vi "Do.vi"(8 "error in (no error)":errorcluster, 10 "Actor in":refnum<class "Actor.lvclass">, 11 "Items Double Click Msg":refnum<class "Items Double Click Msg.lvclass">) -> (0 "error out":errorcluster, 2 "Actor out":refnum<class "Actor.lvclass">)   [LabVIEW 2016, in "Items Double Click Msg.lvclass"]
doc: "This VI delivers the message to the actor by calling the appropriate method(s) on the actor."
uses:
  Items Double Click Msg.lvclass
  <vilib>/ActorFramework/Actor/Actor.lvclass
  Sequence Element/Sequence Element.lvclass
  D:/Program Files/National Instruments/LabVIEW 2016/vi.lib/ActorFramework/Actor/Actor.lvclass
  Items Double Click Msg.lvclass/Items Double Click Msg.ctl
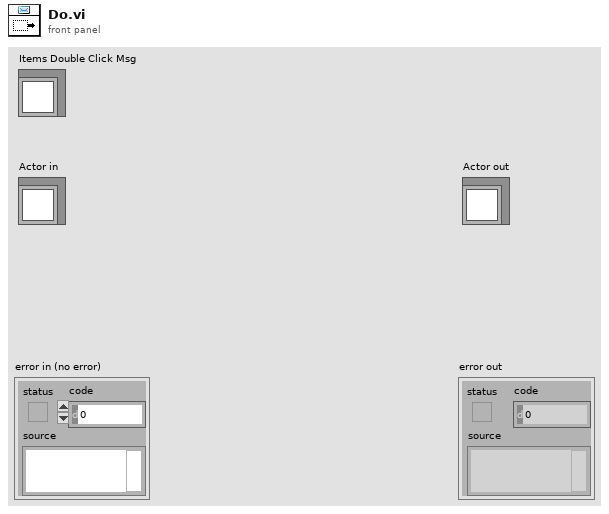
[diagram p1: front panel]
types:
  T1 = typedef "LVPoint32TypeDef.ctl" = cluster{"Horizontal":i32, "Vertical":i32}
  T2 = cluster{"Shift":bool, "Ctrl":bool, "Alt":bool, "Cmd":bool, "Opt":bool}
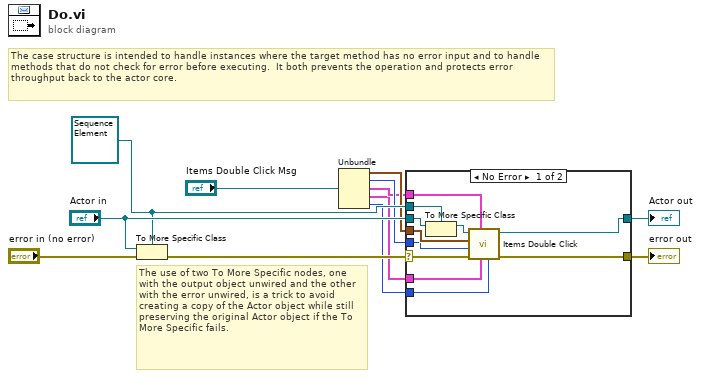
[diagram p0: block diagram]
diagram:
  w6 = refnum<class "Sequence Element.lvclass"> refnum ("Actor in")
  # "The use of two To More Specific nodes, one with the output object unwired and the other with the error unwired, is a trick to avoid creating a copy of the Actor object while still preserving the original Actor object if the To More Specific fails."
  # "The case structure is intended to handle instances where the target method has no error input and to handle methods that do not check for error before executing.  It both prevents the operation and protects error throughput back to the actor core."
  n1 = To More Specific Class(target class=w6, reference="Actor in", error in="error in (no error)") -> (error out=w10:errorcluster)  [unwired: 1 out]
  n2 = Unbundle("Items Double Click Msg") -> (w5:T1, w4:u16, w3:cluster{"Double Click":bool, "Menu Key":bool}, w2:T2, w1:i32)
  n3 = case shown="No Error" w10 {
    selector: w10 -> [w21 w25]
    tunnel: [w23 w25] -> w9
    tunnel: [w22 w24] -> w8
    tunnel: "Actor in" -> [w20 w24]
    tunnel: w6 -> [w19 _]
    tunnel: w5 -> [w17 _]
    tunnel: w4 -> [w16 _]
    tunnel: w3 -> [w15 _]
    tunnel: w2 -> [w14 _]
    tunnel: w1 -> [w13 _]
    frame No Error {
      n4 = To More Specific Class(target class=w19, reference=w20) -> (specific class reference=w18:refnum<class "Sequence Element.lvclass">)  [unwired: 1 in, 1 out]
      n5 = call-dynamic "Items Double Click.vi"("Row"=w13, "PlatMods"=w14, "Mods"=w15, "error in (no error)"=w21, "Button"=w16, "Coords"=w17, "Sequence Element in"=w18) -> ("error out"=w23:errorcluster, "Sequence Element out"=w22:refnum<class "Sequence Element.lvclass">)  [unwired: 3 in]
    }
    frame Error {
      # "If type check fails, pass the original object out again."
    }
  }
  "error out" <- w9
  "Actor out" <- w8
